vi "Out_of_Position.vi"(8 "error in (no error)":errorcluster, 9 "Car Wash Indicators":refnum<vi>, 10 "System data":T1, 11 "Timer":refnum<user-event>) -> (0 "error out":errorcluster, 3 "System data out":T1)   [LabVIEW 2023]
uses:
  Controls/System_Data.ctl
  Controls/Wash Options.ctl
  Controls/State.ctl
  Controls/User_Event.ctl
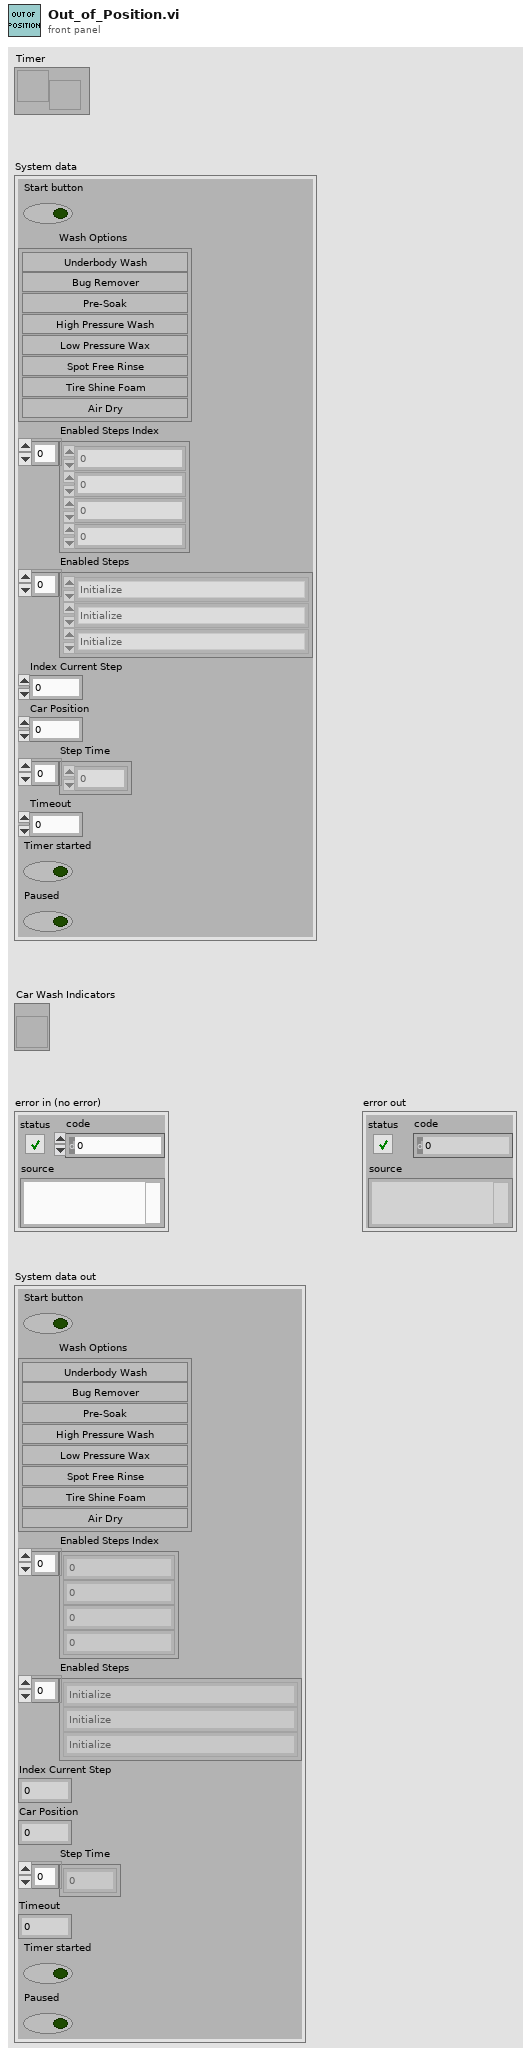
[diagram p1: front panel]
types:
  T1 = typedef "System_Data.ctl" = cluster{"Start button":bool, "Wash Options":T2, "Enabled Steps Index":i32[], "Enabled Steps ":T3[], "Index Current Step":i32, "Car Position":u8, "Step Time":dbl[], "Timeout":i32, "Timer started":bool, "Paused":bool}
  T2 = typedef "Wash Options.ctl" = cluster{"Underbody Wash":bool, "Bug Remover":bool, "Pre-Soak":bool, "High Pressure Wash":bool, "Low Pressure Wax":bool, "Spot Free Rinse":bool, "Tire Shine Foam":bool, "Air Dry":bool}
  T3 = typedef "State.ctl" = enum16{"Initialize", "Wait for Something", "Step Completed", "Save Wash Options", "Start Process", "Car Position", "Order Steps to follow", "Underbody Wash", "Bug Remover", "Pre-Soak", "High Pressure Wash", "Low Pressure Wax", "Spot Free Rinse", "Tire Shine Foam", "Air Dry", "Vehicle out of position", "Exit", "Process Complete", "Stop Application"}
  T4 = typedef "Car Wash Indicators.ctl" = cluster{"Under Body Wash":bool, "Bug Remover":bool, "Pre-Soak":bool, "High Pressure Wash":bool, "Low Pressure Wax":bool, "Spot Free Rinse":bool, "Tire Shine Foam":bool, "Air Dry":bool, "Vehicle Out of Position":bool}
  T5 = typedef "User_Event.ctl" = cluster{"Step Time":dbl, "Timeout":i32, "Pause":bool}
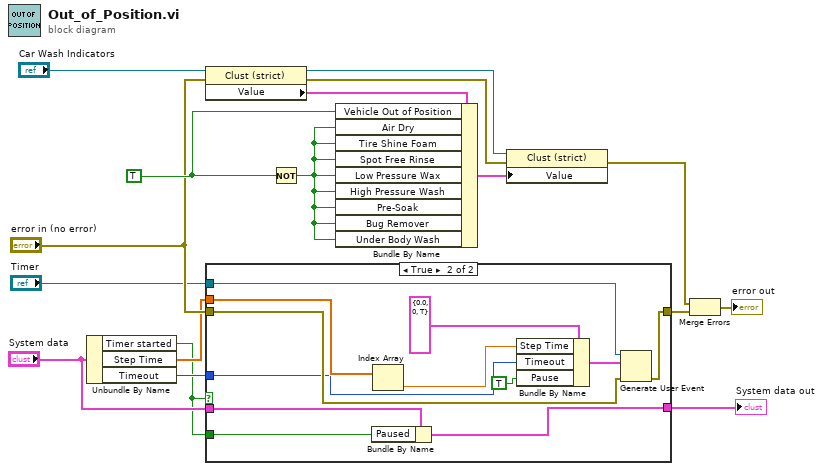
[diagram p0: block diagram]
diagram:
  w16 = TRUE ("Vehicle Out of Position")
  n1 = Unbundle By Name("System data") -> ("Timer started"=w2:bool, "Step Time"=w5:dbl[], "Timeout"=w4:i32)
  n2 = property class="Clust (strict)"(reference="Car Wash Indicators", error in="error in (no error)") -> (reference out=w13:refnum<vi>, error out=w10:errorcluster, "Value"=w14:T4)
  n3 = case shown="True" w2 {
    tunnel: "error in (no error)" -> [w19 w31]
    tunnel: [w19 w29] -> w7
    tunnel: "Timer" -> [_ w30]
    tunnel: w5 -> [_ w25]
    tunnel: w4 -> [_ w24]
    tunnel: "System data" -> [w18 w23]
    tunnel: w2 -> [_ w22]
    tunnel: [w18 w21] -> w1
    frame False {
    }
    frame True {
      n4 = Bundle By Name(cluster=w23, "Paused"=w22) -> (w21:T1)
      n5 = Index Array(array=w25) -> (element=w26:dbl)  [unwired: 1 in]
      n6 = Bundle By Name(cluster=T5 {"Step Time"=0.0, "Timeout"=0, "Pause"=TRUE} ("event data"), "Step Time"=w26, "Timeout"=w24, "Pause"=TRUE) -> (w27:T5)
      n7 = Generate User Event(user event=w30, event data cluster=w27, error in=w31) -> (error out=w29:errorcluster)  [unwired: 1 in, 1 out]
    }
  }
  "System data out" <- w1
  n8 = Not(x=w16) -> (.not. x?=w17:bool)
  n9 = Bundle By Name(cluster=w14, "Vehicle Out of Position"=w16, "Air Dry"=w17, "Tire Shine Foam"=w17, "Spot Free Rinse"=w17, "Low Pressure Wax"=w17, "High Pressure Wash"=w17, "Pre-Soak"=w17, "Bug Remover"=w17, "Under Body Wash"=w17) -> (w15:T4)
  n10 = property class="Clust (strict)"(reference=w13, error in=w10, "Value"=w15) -> (error out=w12:errorcluster)  [unwired: 1 out]
  n11 = Merge Errors(w12, w7) -> (→"error out":errorcluster)
